vi "Planet_Analysis.vi"(8 "error in (no error)":errorcluster, 11 "Conf":T1) -> (0 "error out":errorcluster)   [LabVIEW 2021]
uses:
  Typedefs/PropertyUserChange.ctl
  Typedefs/DataToUserInterface.ctl
  <vilib>/event_ctls.llb/usereventprio.ctl
  <vilib>/Analysis/NI_AALBase.lvlib
  Typedefs/DataToRef.ctl
  Typedefs/State_OA.ctl
  Typedefs/Axis.ctl
  Typedefs/OrderAnalysis.ctl
  Typedefs/Start_End.ctl
  Typedefs/PropertiesOrderAnalysis.ctl
  Typedefs/Detected peaks.ctl
  Typedefs/MeassurementMode.ctl
  Typedefs/PropertiesRead_TDM.ctl
  Typedefs/All_Queues.ctl
  Typedefs/ConfCluster.ctl
  Typedefs/PlanetInfo.ctl
  Typedefs/AllDataToAnal.ctl
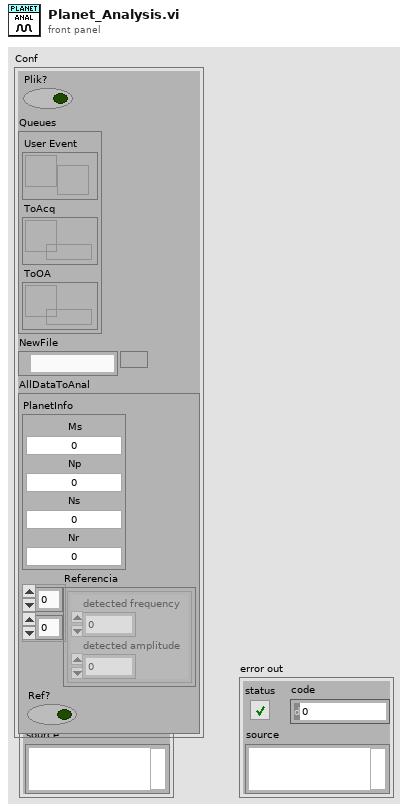
[diagram p1: front panel]
types:
  T1 = typedef "ConfCluster.ctl" = cluster{"Plik?":bool, "Queues":T2, "NewFile":path, "AllDataToAnal":T3}
  T2 = typedef "All_Queues.ctl" = cluster{"User Event":refnum<user-event>, "ToAcq":refnum<queue>, "ToOA":refnum<queue>}
  T3 = typedef "AllDataToAnal.ctl" = cluster{"PlanetInfo":T4, "Referencia":T5[][], "Ref?":bool}
  T4 = typedef "PlanetInfo.ctl" = cluster{"Ms":dbl, "Np":dbl, "Ns":dbl, "Nr":dbl}
  T5 = typedef "Detected peaks.ctl" = cluster{"detected frequency":dbl, "detected amplitude":dbl}
  T6 = typedef "PropertiesOrderAnalysis.ctl" = cluster{"Start/End":T7, "data":waveform(dbl)[], "OrderAnalysis":T8, "Tacho":waveform(dbl)[]}
  T7 = typedef "Start_End.ctl" = enum16{"Start", "End"}
  T8 = typedef "OrderAnalysis.ctl" = cluster{"dB on":bool, "window type":u32, "max order to analyze":dbl, "order resolution":dbl, "Axis":T9, "Sample rate":i64, "Save?":bool, "Multiple_Frequency":i32, "averaging mode":enum16{"No averaging", "Vector averaging", "RMS averaging", "Peak hold"}}
  T9 = typedef "Axis.ctl" = u16
  T10 = typedef "State_OA.ctl" = enum16{"Wait", "Init", "Show", "Save"}
  T11 = typedef "usereventprio.ctl" = enum32{"high priority", "normal priority"}
  T12 = typedef "PropertyUserChange.ctl" = enum16{"Default", "Results", "Start", "Save", "CanalNames"}
  T13 = typedef "DataToUserInterface.ctl" = cluster{"Value":variant, "Property":T12}
  T14 = typedef "DataToRef.ctl" = cluster{"NumberOfEl":dbl, "Freq_Ch1":dbl[], "Amp_Ch1":dbl[], "Freq_Ch2":dbl[], "Amp_Ch2":dbl[], "Freq_Ch3":dbl[], "Amp_Ch3":dbl[]}
  T15 = enum16{"open", "open or create", "create or replace", "create", "open (read-only)"}
  T16 = typedef "DataToUI.ctl" = cluster{"Speed profile":cluster{"time [s]":dbl[], "speed [RPM]":dbl[]}, "Results":T17[], "Vibration signals":waveform(dbl)[]}
  T17 = typedef "Results.ctl" = cluster{"Power Spectrum / PSD":cluster{"f0":dbl, "df":dbl, "magnitude":dbl[]}[], "Order power spectra":cluster{"order 0":dbl, "delta order":dbl, "magnitude":dbl[]}[], "Actual max order":dbl, "Mesh_Freq":dbl[], "Detected peaks":T5[][], "Alarm?":bool[], "Exceed":string[][], "Mesh_mean":dbl, "Mesh_std":dbl}
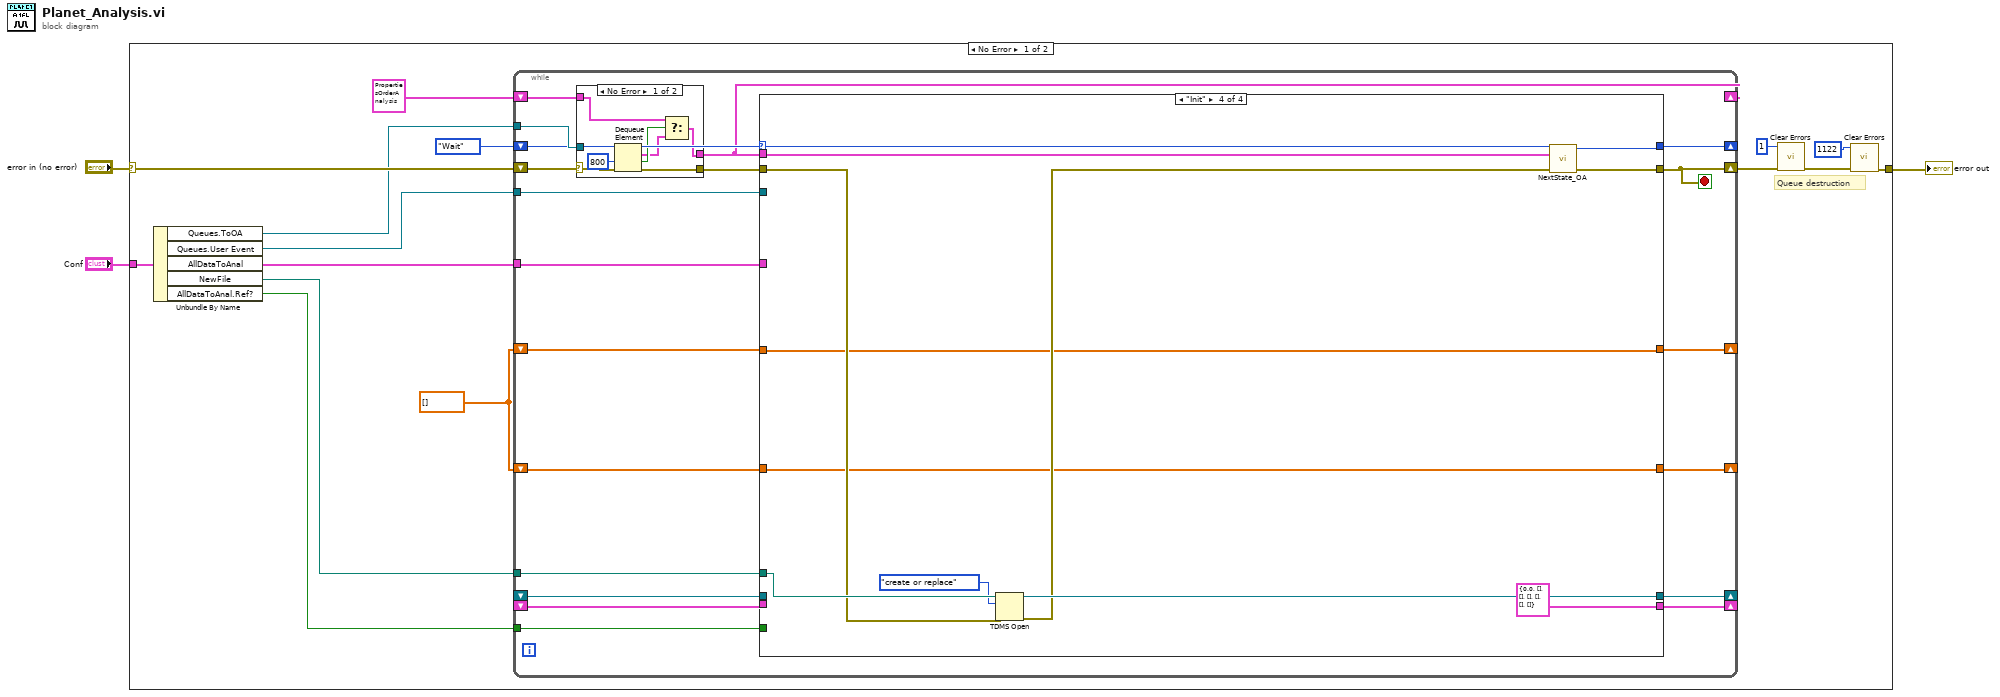
[diagram p0: block diagram]
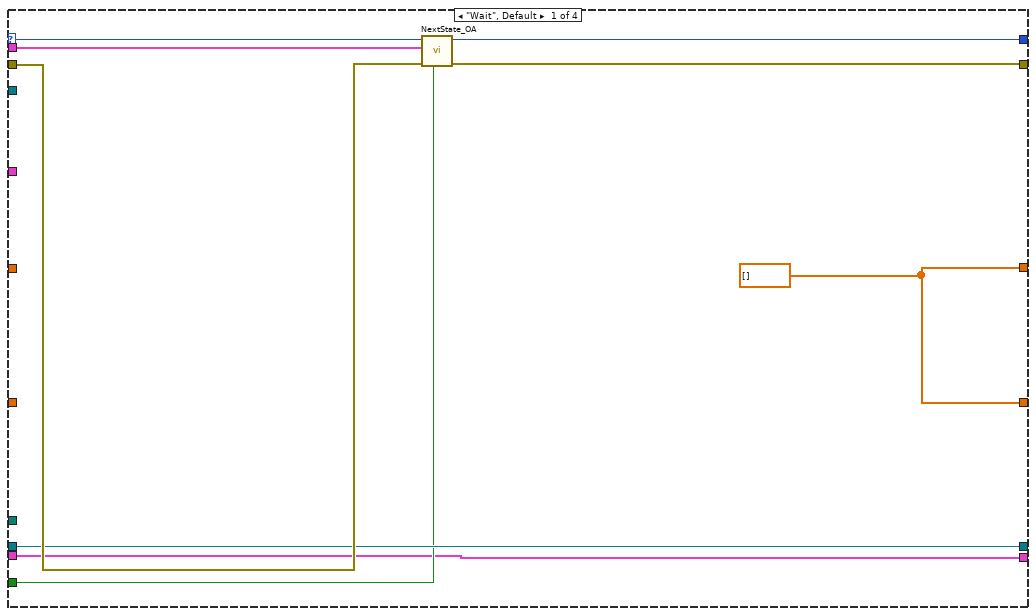
[diagram p2: hidden frame]
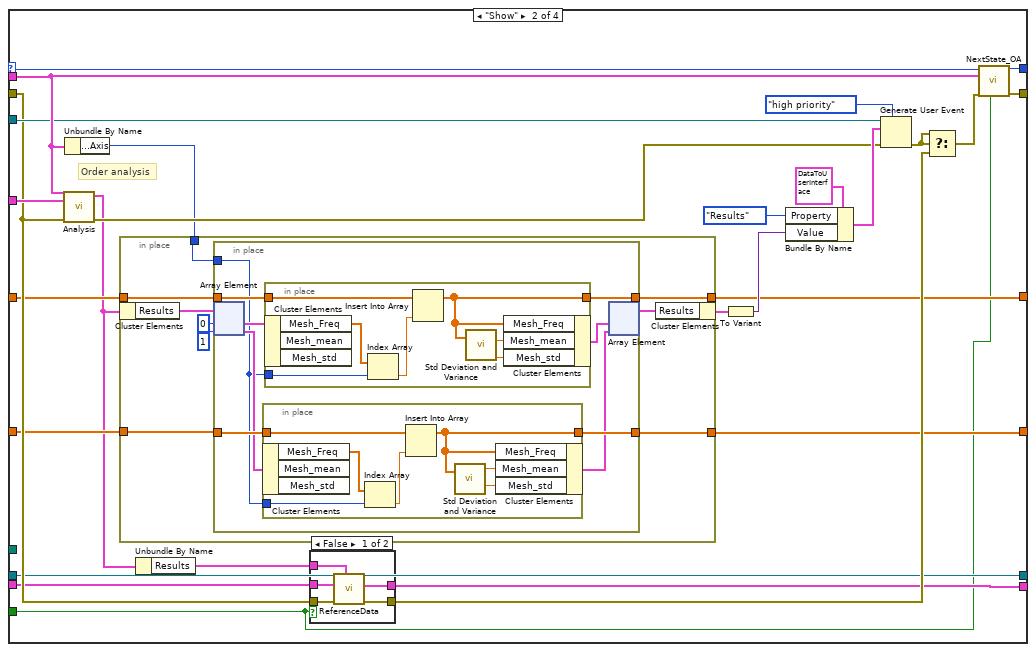
[diagram p3: hidden frame]
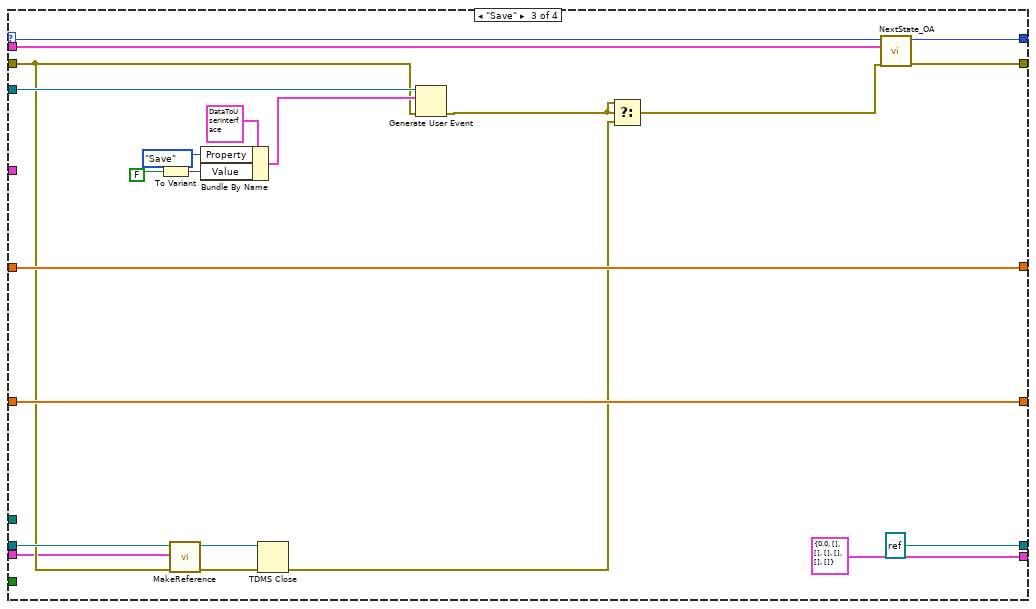
[diagram p5: hidden frame]
diagram:
  n1 = case shown="No Error" "error in (no error)" {
    selector: "error in (no error)" -> [w17 w159]
    tunnel: [w18 w159] -> w3
    tunnel: "Conf" -> [w11 _]
    frame No Error {
      w10 = dbl[] []
      # "Queue destruction"
      n2 = Unbundle By Name(w11) -> ("Queues.ToOA"=w12:refnum<queue>, "Queues.User Event"=w13:refnum<user-event>, "AllDataToAnal"=w14:T3, "NewFile"=w16:path, "AllDataToAnal.Ref?"=w15:bool)
      n3 = while {
        tunnel: w12 -> [w35]
        shift-right: [w38] -> w7
        shift-left: w17 -> [w37]
        shift-right: [w32] -> _
        shift-left: T6 {"Start/End"=enum."End", "data"=[], "OrderAnalysis"={"dB on"=TRUE, "window type"=1, "max order to analyze"=32.0, "order resolution"=0.1, "Axis"=0, "Sample rate"=5000, "Save?"=FALSE, "Multiple_Frequency"=3, "averaging mode"=enum."No averaging"}, "Tacho"=[]} -> [w36]
        shift-right: [w31] -> _
        shift-left: State_OA."Wait" -> [w33]
        shift-right: [w30] -> _
        shift-left: w10 -> [w29]
        shift-right: [w28] -> _
        shift-left: w10 -> [w27]
        tunnel: w13 -> [w26]
        shift-right: [w25] -> _
        shift-left: _ -> [w24]
        tunnel: w14 -> [w23]
        tunnel: w15 -> [w22]
        tunnel: w16 -> [w21]
        shift-right: [w20] -> _
        shift-left: _ -> [w19]
        stop <- w38 stop-if-true
        n4 = case shown="No Error" w37 {
          selector: w37 -> [w153 w158]
          tunnel: [w154 w158] -> w34
          tunnel: [w151 w157] -> w32
          tunnel: w35 -> [w150 _]
          tunnel: w36 -> [w149 w157]
          frame No Error {
            n5 = Dequeue Element(queue=w150, timeout in ms (-1)=800, error in (no error)=w153) -> (element=w152:T6, timed out?=w156:bool, error out=w154:errorcluster)  [unwired: 1 out]
            n6 = Select(t=w149, s=w156, f=w152) -> (s? t:f=w151:T6)
          }
          frame Error {
          }
        }
        n7 = case shown="\"Init\"" w33 {
          selector: w33 -> [w44 w73 w134 w143]
          tunnel: [w46 w75 w132 w140] -> w38
          tunnel: w34 -> [w42 w60 w117 w146]
          tunnel: w32 -> [w47 w72 w131 w142]
          tunnel: [w45 w74 w133 w144] -> w31
          tunnel: [w43 w53 w135 w138] -> w30
          tunnel: w29 -> [_ w54 w135 w138]
          tunnel: [w43 w52 w136 w139] -> w28
          tunnel: w27 -> [_ w55 w136 w139]
          tunnel: w26 -> [_ w66 w127 _]
          tunnel: [w41 w59 refnum<k34> refnum ("tdms file out") w147] -> w25
          tunnel: w24 -> [w41 w59 w118 _]
          tunnel: w23 -> [_ w62 _ _]
          tunnel: w22 -> [w40 w48 _ _]
          tunnel: w21 -> [_ _ _ w148]
          tunnel: [w39 w58 T14 {"NumberOfEl"=0.0, "Freq_Ch1"=[], "Amp_Ch1"=[], "Freq_Ch2"=[], "Amp_Ch2"=[], "Freq_Ch3"=[], "Amp_Ch3"=[]} ("DatatoRef out") T14 {"NumberOfEl"=0.0, "Freq_Ch1"=[], "Amp_Ch1"=[], "Freq_Ch2"=[], "Amp_Ch2"=[], "Freq_Ch3"=[], "Amp_Ch3"=[]} ("DatatoRef out")] -> w20
          tunnel: w19 -> [w39 w57 w115 _]
          frame "Wait", Default {
            w43 = dbl[] []
            n8 = call "NextState_OA.vi"("Ref?"=w40, "error in (no error)"=w42, "Prop"=w47, "Previous Step"=w44) -> ("error out"=w46:errorcluster, "Next Step"=w45:T10)  [unwired: 6 in]
          }
          frame "Show" {
            # "Order analysis"
            n9 = call "Analysis.vi"("error in (no error)"=w60, "AllDataToAnal"=w62, "PropertiesToOrderAnalysis"=w72) -> ("error out"=w67:errorcluster, "DataToUI"=w50:T16)  [unwired: 7 in]
            n10 = Unbundle By Name(w72) -> ("OrderAnalysis.Axis"=w56:T9)
            n11 = in-place {
              in-place-border: w56 -> [w81]
              in-place-border: w55 -> [w80]
              in-place-border: w54 -> [w79]
              in-place-border: [w78] -> w53
              in-place-border: [w77] -> w52
              n12 = in-place-cluster #1(w50) -> ("Results"=w76:T17[])
              n13 = in-place {
                in-place-border: w80 -> [w93]
                in-place-border: w81 -> [w88]
                in-place-border: [w92] -> w77
                in-place-border: w79 -> [w90]
                in-place-border: [w87] -> w78
                n14 = in-place-array #2(w76, 0, 1) -> (w91:T17, w89:T17)
                n15 = in-place {
                  in-place-border: w90 -> [w100]
                  in-place-border: [w96] -> w87
                  in-place-border: w88 -> [w97]
                  n16 = in-place-cluster #3(w89) -> ("Mesh_Freq"=w99:dbl[])  [unwired: 2 out]
                  n17 = Index Array(array=w99, index=w97) -> (element=w98:dbl)
                  n18 = Insert Into Array(array=w100, new element=w98) -> (w96:dbl[])  [unwired: 1 in]
                  n19 = call <vilib>:"Std Deviation and Variance.vi"("X"=w96) -> ("mean"=w95:dbl, "standard deviation"=w94:dbl)  [unwired: 1 in, 1 out]
                  n20 = in-place-cluster #3("Mesh_Freq"=w96, "Mesh_mean"=w95, "Mesh_std"=w94) -> (w85:T17)
                }
                n21 = in-place {
                  in-place-border: w93 -> [w107]
                  in-place-border: w88 -> [w106]
                  in-place-border: [w103] -> w92
                  n22 = in-place-cluster #4(w91) -> ("Mesh_Freq"=w105:dbl[])  [unwired: 2 out]
                  n23 = Index Array(array=w105, index=w106) -> (element=w104:dbl)
                  n24 = Insert Into Array(array=w107, new element=w104) -> (w103:dbl[])  [unwired: 1 in]
                  n25 = call <vilib>:"Std Deviation and Variance.vi"("X"=w103) -> ("mean"=w102:dbl, "standard deviation"=w101:dbl)  [unwired: 1 in, 1 out]
                  n26 = in-place-cluster #4("Mesh_Freq"=w103, "Mesh_mean"=w102, "Mesh_std"=w101) -> (w86:T17)
                }
                n27 = in-place-array #2(w86, w85) -> (w82:T17[])  [unwired: 2 out]
              }
              n28 = in-place-cluster #1("Results"=w82) -> (w51:T16)
            }
            n29 = Unbundle By Name(w50) -> ("Results"=w49:T17[])
            n30 = case shown="False" w48 {
              tunnel: [w112 w114] -> w61
              tunnel: w60 -> [w111 w114]
              tunnel: [w110 w113] -> w58
              tunnel: w57 -> [w109 w113]
              tunnel: w49 -> [w108 _]
              frame False {
                n31 = call "ReferenceData.vi"("Results"=w108, "error in (no error)"=w111, "DatatoRef in"=w109) -> ("error out"=w112:errorcluster, "DatatoRef out"=w110:T14)  [unwired: 7 in]
              }
              frame True {
              }
            }
            n32 = To Variant(anything=w51) -> (Variant=w68:variant)
            n33 = Bundle By Name(cluster=T13 {"Value"=variant, "Property"=enum."Default"} ("UserData"), "Property"=PropertyUserChange."Results", "Value"=w68) -> (w70:T13)
            n34 = Generate User Event(priority (normal)=usereventprio."high priority", user event=w66, event data cluster=w70, error in=w67) -> (error out=w64:errorcluster)  [unwired: 1 out]
            n35 = Select(t=w64, s=w64, f=w61) -> (s? t:f=w63:errorcluster)
            n36 = call "NextState_OA.vi"("Ref?"=w48, "error in (no error)"=w63, "Prop"=w72, "Previous Step"=w73) -> ("error out"=w75:errorcluster, "Next Step"=w74:T10)  [unwired: 6 in]
          }
          frame "Save" {
            n37 = To Variant(anything=FALSE) -> (Variant=w128:variant)
            n38 = call "MakeReference.vi"("error in (no error)"=w117, "DatatoRef"=w115, "Refnum in"=w118) -> ("error out"=w119:errorcluster, "Refnum out"=w120:refnum<k34>)  [unwired: 7 in]
            n39 = Bundle By Name(cluster=T13 {"Value"=variant, "Property"=enum."Default"} ("UserData"), "Property"=PropertyUserChange."Save", "Value"=w128) -> (w126:T13)
            n40 = TDMS Close(8:w119, 11:w120) -> (0:w122:errorcluster)  [unwired: 1 out]
            n41 = Generate User Event(user event=w127, event data cluster=w126, error in=w117) -> (error out=w123:errorcluster)  [unwired: 1 in, 1 out]
            n42 = Select(t=w123, s=w123, f=w122) -> (s? t:f=w121:errorcluster)
            n43 = call "NextState_OA.vi"("error in (no error)"=w121, "Prop"=w131, "Previous Step"=w134) -> ("error out"=w132:errorcluster, "Next Step"=w133:T10)  [unwired: 7 in]
          }
          frame "Init" {
            n44 = TDMS Open(8:w146, 10:T15."create or replace" ("operation (0:open)"), 11:w148) -> (0:w141:errorcluster, 3:w147:refnum<k34>)  [unwired: 4 in]
            n45 = call "NextState_OA.vi"("error in (no error)"=w141, "Prop"=w142, "Previous Step"=w143) -> ("error out"=w140:errorcluster, "Next Step"=w144:T10)  [unwired: 7 in]
          }
        }
      }
      n46 = call <vilib>:"Clear Errors.vi"("error in (no error)"=w7, "specific error code to clear (0: all)"=1) -> ("error out"=w5:errorcluster)  [unwired: 4 in, 1 out]
      n47 = call <vilib>:"Clear Errors.vi"("error in (no error)"=w5, "specific error code to clear (0: all)"=1122) -> ("error out"=w18:errorcluster)  [unwired: 4 in, 1 out]
    }
    frame Error {
    }
  }
  "error out" <- w3
